vi "SetImageBuffer.vi"(8 "error in (no error)":errorcluster, 10 "max queue size (-1, unlimited)":i32, 11 "Camera in":refnum<class "Camera.lvclass">) -> (0 "error out":errorcluster, 3 "Camera out":refnum<class "Camera.lvclass">)   [LabVIEW 2020, in "Camera.lvlib" / "Camera.lvclass"]
uses:
  Camera.lvclass
  <vilib>/vision/Image Controls.llb/IMAQ Image.ctl
  Camera.lvclass/Camera.ctl
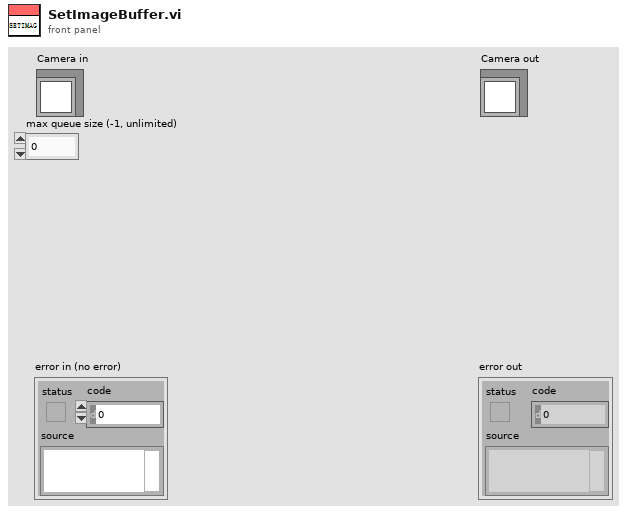
[diagram p1: front panel]
types:
  T1 = typedef "IMAQ Image.ctl" = refnum<image>
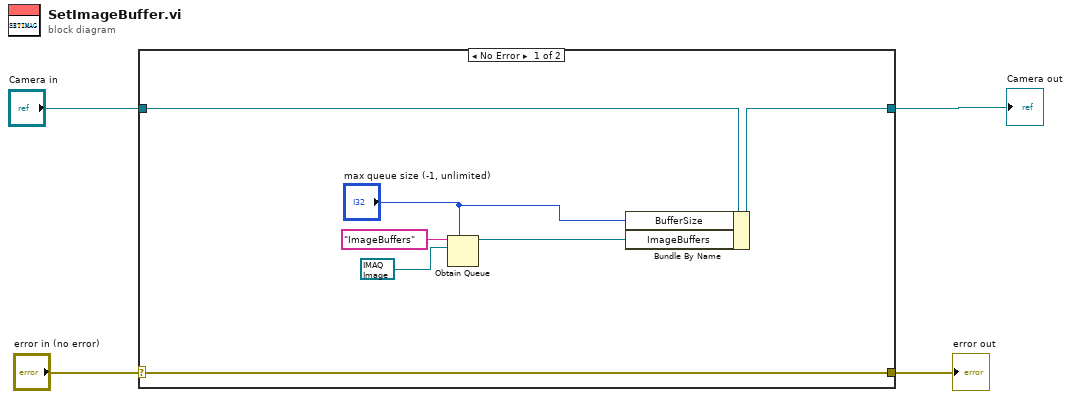
[diagram p0: block diagram]
diagram:
  n1 = case shown="No Error" "error in (no error)" {
    selector: "error in (no error)" -> [w11 w13]
    tunnel: [w11 w13] -> w3
    tunnel: [w9 w12] -> w1
    tunnel: "Camera in" -> [w10 w12]
    frame No Error {
      n2 = Obtain Queue(max queue size (-1, unlimited)="max queue size (-1, unlimited)", name (unnamed)="ImageBuffers", element data type=T1 refnum ("New Image")) -> (queue out=w8:refnum<queue>)  [unwired: 2 in, 2 out]
      n3 = Bundle By Name(cluster=w10, "BufferSize"="max queue size (-1, unlimited)", "ImageBuffers"=w8) -> (w9:refnum<class "Camera.lvclass">)
    }
    frame Error {
    }
  }
  "error out" <- w3
  "Camera out" <- w1
